vi "температура азот.vi"(11 "Температура":dbl) -> (3 "вязкость":dbl)   [LabVIEW 2018]
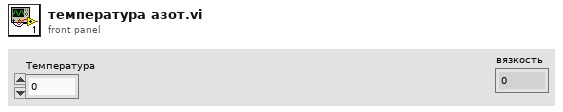
[diagram p1: front panel]
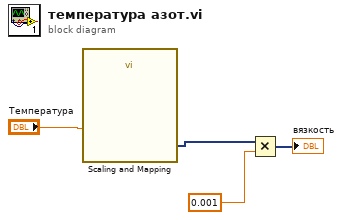
[diagram p0: block diagram]
diagram:
  n1 = call "Scaling and Mapping"("Signals"="Температура") -> ("Scaled Signals"=w3:dynamicdata)  [unwired: 9 in, 1 out]
  n2 = Multiply(x=w3, y=0.001) -> (x*y=→"вязкость":dynamicdata)
